vi "Initialize.vi"(8 "error in (no error)":errorcluster, 10 "Top Level Diagram":refnum<vi>, 11 "Initial Sequence in":refnum<class "Main Sequence.lvclass">) -> (0 "error out":errorcluster, 3 "Initial Sequence out":refnum<class "Main Sequence.lvclass">)   [LabVIEW 2015, in "Main Sequence.lvclass"]
uses:
  Main Sequence.lvclass
  <vilib>/Utility/miscctls.llb/LVPointTypeDef.ctl
  Structures/Structures.lvclass/Structures.ctl
  Structures/Write Structure.vi
  Structures/Write Diagram.vi
  Structures/Write Location.vi
  Structures/Structures.lvclass
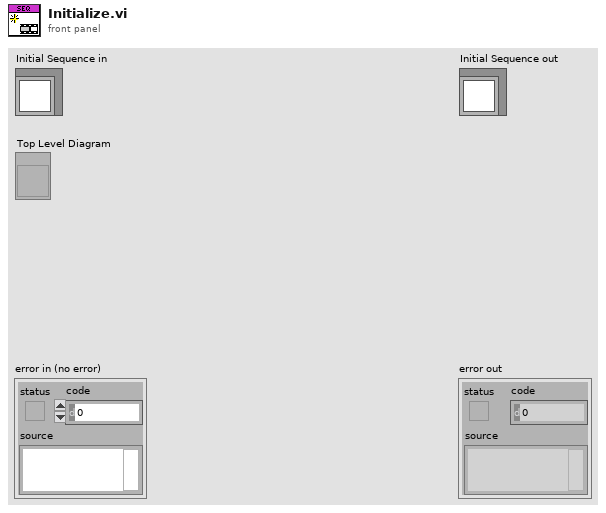
[diagram p1: front panel]
types:
  T1 = typedef "LVPointTypeDef.ctl" = cluster{"Horizontal":i16, "Vertical":i16}
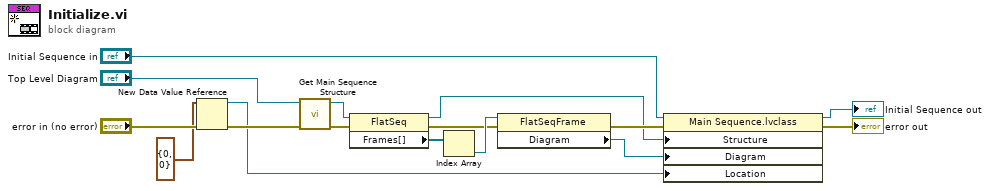
[diagram p0: block diagram]
diagram:
  n1 = New Data Value Reference(data value=T1 {"Horizontal"=0, "Vertical"=0} ("location out"), error in="error in (no error)") -> (data value reference=w1:refnum<data-value>, error out=w3:errorcluster)
  n2 = call "Get Main Sequence Structure.vi"("error in (no error)"=w3, "Top Level Diagram"="Top Level Diagram") -> ("error out"=w15:errorcluster, "Main.SeqStructure"=w14:refnum<vi>)  [unwired: 8 in]
  n3 = property class="FlatSeq"(reference=w14, error in=w15) -> (reference out=w5:refnum<vi>, error out=w12:errorcluster, "Frames[]"=w16:refnum<vi>[])
  n4 = Index Array(array=w16) -> (element=w13:refnum<vi>)  [unwired: 1 in]
  n5 = property class="FlatSeqFrame"(reference=w13, error in=w12) -> (error out=w11:errorcluster, "Diagram"=w6:refnum<vi>)  [unwired: 1 out]
  n6 = property class="Main Sequence.lvclass"(reference="Initial Sequence in", error in=w11, "Structure"=w5, "Diagram"=w6, "Location"=w1) -> (reference out=→"Initial Sequence out":refnum<class "Main Sequence.lvclass">, error out=→"error out":errorcluster)
